vi "Get ImageDataAsPicture.vi"(8 "error in (no error)":errorcluster, 10 "GetElement (-1: Current)":i32=-1, 11 "CircularBuffer.ImageData":refnum<class "CircularBuffer.ImageData.lvclass">) -> (0 "error out":errorcluster, 2 "Selected Image":picture, 3 "CircularBuffer.ImageData out":refnum<class "CircularBuffer.ImageData.lvclass">)   [LabVIEW 2013, in "CircularBuffer.ImageData.lvclass"]
uses:
  CircularBuffer.ImageData.lvclass
  CircularBuffer/CircularBuffer.lvclass
  <vilib>/picture/picture.llb/imagedata.ctl
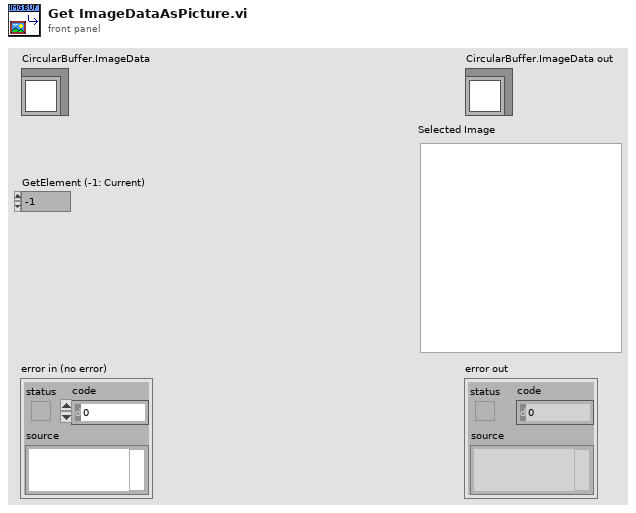
[diagram p1: front panel]
types:
  T1 = typedef "imagedata.ctl" = cluster{"image type":i32, "image depth":i32, "image":u8[], "mask":u8[], "colors":u32[], "Rectangle":cluster{"left":i16, "top":i16, "right":i16, "bottom":i16}}
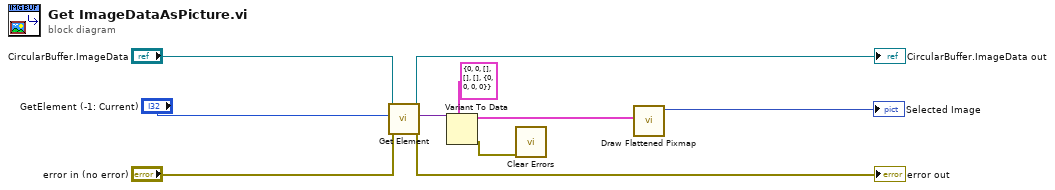
[diagram p0: block diagram]
diagram:
  n1 = call "Get Element.vi"("error in (no error)"="error in (no error)", "GetElement (-1: Current)"="GetElement (-1: Current)", "CircularBuffer"="CircularBuffer.ImageData") -> ("error out"=→"error out":errorcluster, "Element"=w5:variant, "CircularBuffer out"=→"CircularBuffer.ImageData out":refnum<class "CircularBuffer.ImageData.lvclass">)  [unwired: 6 in]
  n2 = Variant To Data(type=T1 {"image type"=0, "image depth"=0, "image"=[], "mask"=[], "colors"=[], "Rectangle"={"left"=0, "top"=0, "right"=0, "bottom"=0}} ("ImageData"), Variant=w5) -> (data=w3:T1, error out=w1:errorcluster)  [unwired: 1 in]
  n3 = call <vilib>:"Clear Errors.vi"("error in (no error)"=w1) -> ()  [unwired: 5 in, 2 out]
  n4 = call <vilib>:"Draw Flattened Pixmap.vi"("image data"=w3) -> ("new picture"=→"Selected Image":picture)  [unwired: 8 in]
